vi "Names Data Set.vi"(0 "Name Actions":T1, 11 "error in (no error)":errorcluster) -> (1 "Actuator Command Volts":string[](array[string])=["Command  X1 (V)", "Command  X2 (V)", "Command  Y1 (V)", "Command  Z1 (V)", "Command  Z2 (V)", "Command  Z3 (V)"], 2 "Actuator Volt Readings":string[](array[string])=["LVDT X1 (V)", "LVDT X2 (V)", "LVDT Y1 (V)", "LVDT Z1 (V)", "LVDT Z2 (V)", "LVDT Z3 (V)", "Load Cell X1 (V)", "Load Cell X2 (V)", "Load Cell Y1 (V)", "Load Cell Z1 (V)", "Load Cell Z2 (V)", "Load Cell Z3 (V)"], 3 "Servo Names":string[](array[string])=["Servo Error X1 (V)", "Servo Error X2 (V)", "Servo Error Y1 (V)", "Servo Error Z1 (V)", "Servo Error Z2 (V)", "Servo Error Z3 (V)"], 4 "Cartesian Commands":string[](array[string])=["CommandDx (in)", "CommandDy (in)", "CommandDz (in)", "CommandRx (rad)", "CommandRy (rad)", "CommandRz (rad)"], 6 "Cartesian Readings":string[](array[string])=["Dx (in)", "Dy (in)", "Dz (in)", "Rx (rad)", "Ry (rad)", "Rz (rad)", " Fx (lbs)", " Fy (lbs)", " Fz (lbs)", " Mx (lb*in)", " My (lb*in)", " Mz (lb*in)"], 8 "Actuator Commands":string[](array[string])=["Command  X1 (in)", "Command  X2 (in)", "Command  Y1 (in)", "Command  Z1 (in)", "Command  Z2 (in)", "Command  Z3 (in)"], 10 "Actuator Readings":string[](array[string])=["LVDT X1 (in)", "LVDT X2 (in)", "LVDT Y1 (in)", "LVDT Z1 (in)", "LVDT Z2 (in)", "LVDT Z3 (in)", "Load Cell X1 (lbs)", "Load Cell X2 (lbs)", "Load Cell Y1 (lbs)", "Load Cell Z1 (lbs)", "Load Cell Z2 (lbs)", "Load Cell Z3 (lbs)"], 13 "External Sensor Names":string[](array[string]), 14 "Cartesian Force Commands":string[](array[string])=["Command Fx (lbs)", "Command Fy (lbs)", "Command Fz (lbs)", "Command Mx (lb*in)", "Command My (lb*in)", "Command Mz (lb*in)"], 15 "error out":errorcluster)   [LabVIEW 2013]
uses:
  Name Actions.ctl
  Data Access Objects/Metadata/Persistant DAO Actions.ctl
  Data Access Objects/Metadata/LBCB Number.ctl
panel:
  in  "Actuators":string[](array[string])=["X1", "X2", "Y1", "Z1", "Z2", "Z3"]
  in  "Cartesian Force":string[](array[string])=["Fx (lbs)", "Fy (lbs)", "Fz (lbs)", "Mx (lb*in)", "My (lb*in)", "Mz (lb*in)"]
  in  "Cartesian Displacement Units":string[](array[string])=["Dx (in)", "Dy (in)", "Dz (in)", "Rx (rad)", "Ry (rad)", "Rz (rad)"]
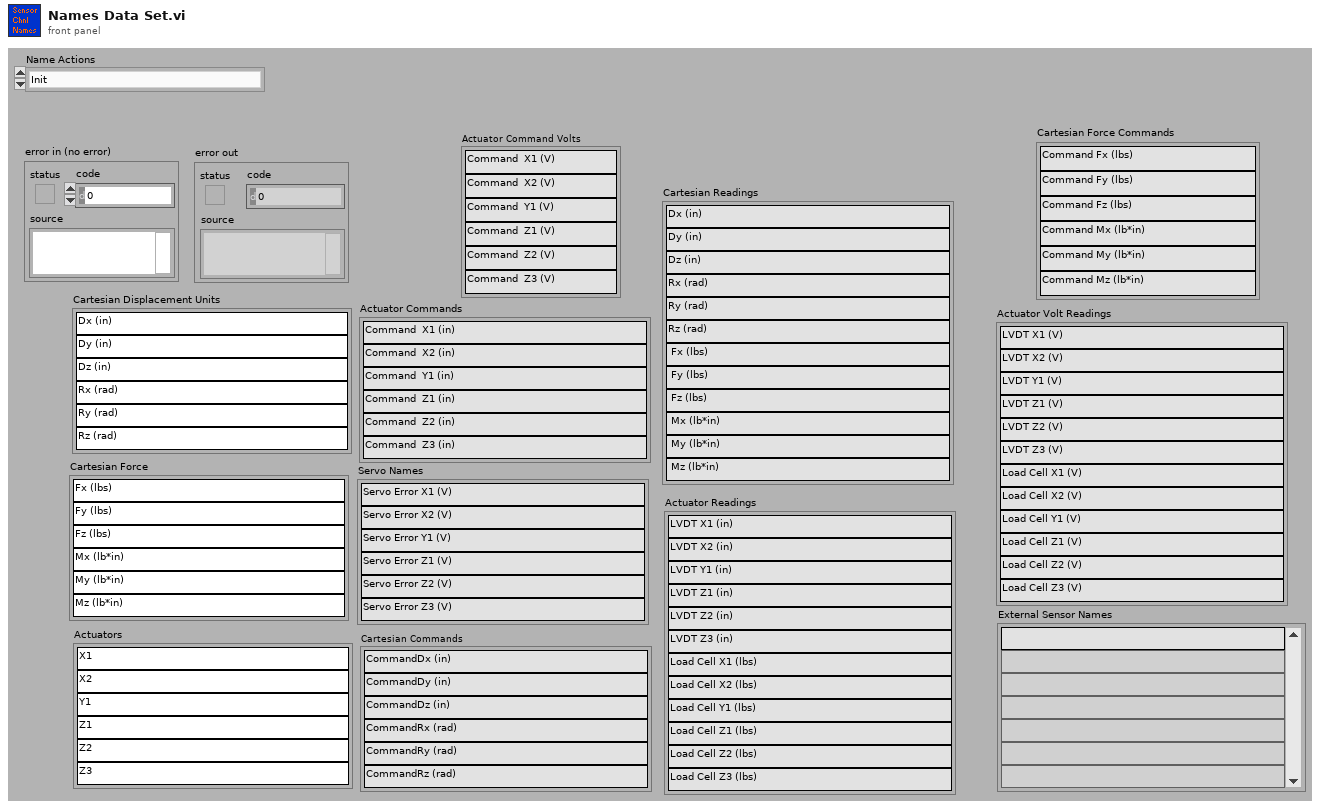
[diagram p1: front panel]
types:
  T1 = typedef "Name Actions.ctl" = enum16{"Init", "Get Names", "Get Index"}
  T2 = typedef "LBCB Number.ctl" = enum16{"LBCB1", "LBCB2"}
  T3 = typedef "Persistant DAO Actions.ctl" = enum16{"Init", "Get", "Set", "Load", "Save"}
  T4 = typedef "LBCB Settings.ctl" = cluster{"Size":T5, "Type":T6}
  T5 = typedef "LBCB Size.ctl" = enum16{"1/5th-scale LBCB", "Full-scale LBCB", "Portable LBCB", "Mid-Scale LBCB"}
  T6 = typedef "LBCB Type.ctl" = enum16{"X Actuators On The Left", "X Actuators On The Right"}
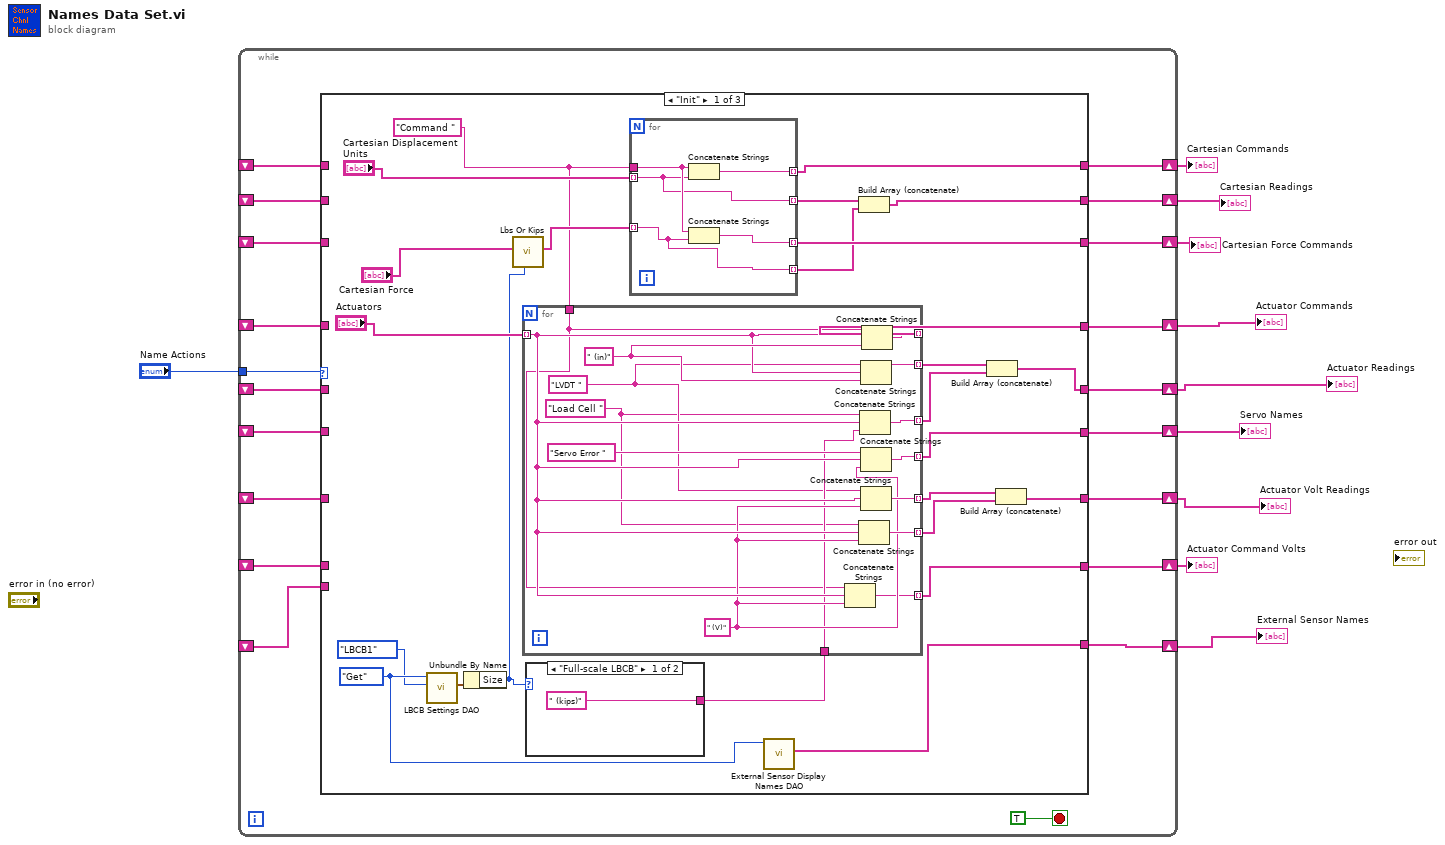
[diagram p0: block diagram]
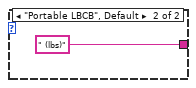
[diagram p2: hidden frame]
diagram:
  n1 = while {
    tunnel: "Name Actions" -> [w29]
    shift-right: [w28] -> w9
    shift-left: _ -> [w24]
    shift-right: [w27] -> w8
    shift-left: _ -> [w22]
    shift-right: [w26] -> w7
    shift-left: _ -> [w23]
    shift-right: [w25] -> w6
    shift-left: _ -> [w21]
    shift-right: [w20] -> w5
    shift-left: _ -> [w19]
    shift-right: [w18] -> w4
    shift-left: _ -> [w17]
    shift-right: [w16] -> w3
    shift-left: _ -> [w15]
    shift-right: [w14] -> w2
    shift-left: _ -> [w13]
    shift-right: [w12] -> w1
    shift-left: _ -> [w11]
    stop <- TRUE stop-if-true
    n2 = case shown="\"Init\"" w29 {
      tunnel: [w48 w86 w95] -> w28
      tunnel: [w43 w84 w93] -> w27
      tunnel: [w42 w85 w94] -> w26
      tunnel: [w41 w83 w92] -> w25
      tunnel: w24 -> [_ w86 w95]
      tunnel: w23 -> [_ w85 w94]
      tunnel: w22 -> [_ w84 w93]
      tunnel: w21 -> [_ w83 w92]
      tunnel: [w47 w82 w91] -> w20
      tunnel: w19 -> [_ w82 w91]
      tunnel: [w45 w81 w90] -> w18
      tunnel: w17 -> [_ w81 w90]
      tunnel: [w46 w80 w89] -> w16
      tunnel: w15 -> [_ w80 w89]
      tunnel: [w44 w79 w88] -> w14
      tunnel: w13 -> [_ w79 w88]
      tunnel: [w40 w78 w87] -> w12
      tunnel: w11 -> [_ w78 w87]
      frame "Init" {
        w38 = Persistant_DAO_Actions."Get" ("Persistent DAO Actions")
        w31 = "Command " ("string")
        n3 = call "LBCB Settings DAO.vi"("LBCB Number"=LBCB_Number."LBCB1", "Actions"=w38) -> ("LBCB Setting Out"=w36:T4)  [unwired: 7 in, 2 out]
        n4 = Unbundle By Name(w36) -> ("Size"=w32:T5)
        n5 = call "Lbs Or Kips.vi"("Size"=w32, "Cartesian Force In"="Cartesian Force") -> ("Cartesian Force In Out"=w33:string[])  [unwired: 9 in]
        n6 = case shown="\"Full-scale LBCB\"" w32 {
          tunnel: [" (kips)" ("string") " (lbs)" ("string")] -> w35
          frame "Full-scale LBCB" {
          }
          frame "Portable LBCB", Default {
          }
        }
        n7 = for {
          tunnel: "Actuators" -> [w64] mode=indexing
          tunnel: [w70] -> w45 mode=indexing
          tunnel: [w69] -> w52 mode=indexing
          tunnel: [w68] -> w51 mode=indexing
          tunnel: [w67] -> w42 mode=indexing
          tunnel: [w66] -> w50 mode=indexing
          tunnel: [w65] -> w49 mode=indexing
          tunnel: [w62] -> w44 mode=indexing
          tunnel: w35 -> [w61]
          tunnel: w31 -> [w58]
          w59 = "Load Cell " ("string")
          w60 = "LVDT " ("string")
          w63 = " (V)" ("string")
          w72 = " (in)" ("string")
          n8 = Concatenate Strings(w58, w64, w63) -> (w62:string)
          n9 = Concatenate Strings(w59, w64, w63) -> (w65:string)
          n10 = Concatenate Strings(w59, w64, w61) -> (w68:string)
          n11 = Concatenate Strings(w60, w64, w72) -> (w69:string)
          n12 = Concatenate Strings("Servo Error " ("string"), w64, w63) -> (w67:string)
          n13 = Concatenate Strings(w60, w64, w63) -> (w66:string)
          n14 = Concatenate Strings(w58, w64, w72) -> (w70:string)
        }
        n15 = for {
          tunnel: w31 -> [w76]
          tunnel: "Cartesian Displacement Units" -> [w74] mode=indexing
          tunnel: [w77] -> w46 mode=indexing
          tunnel: [w74] -> w54 mode=indexing
          tunnel: w33 -> [w73] mode=indexing
          tunnel: [w75] -> w40 mode=indexing
          tunnel: [w73] -> w39 mode=indexing
          n16 = Concatenate Strings(w76, w74) -> (w77:string)
          n17 = Concatenate Strings(w76, w73) -> (w75:string)
        }
        n18 = call "External Sensor Display Names DAO.vi"("Persistent DAO Actions"=w38) -> ("Display Name Out"=w41:string[])  [unwired: 3 in, 7 out]
        n19 = Build Array (concatenate)(w54, w39) -> (w48:string[])
        n20 = Build Array (concatenate)(w52, w51) -> (w47:string[])
        n21 = Build Array (concatenate)(w50, w49) -> (w43:string[])
      }
      frame "Get Names" {
      }
      frame "Get Index" {
      }
    }
  }
  "Cartesian Readings" <- w9
  "Actuator Volt Readings" <- w8
  "Servo Names" <- w7
  "External Sensor Names" <- w6
  "Actuator Readings" <- w5
  "Actuator Commands" <- w4
  "Cartesian Commands" <- w3
  "Actuator Command Volts" <- w2
  "Cartesian Force Commands" <- w1
